vi "Main.vi"() -> ()   [LabVIEW 2017]
uses:
  CTL/REF Channel Select.ctl
  D:/test/ILSTS/LV_IL/LV_IL_Sample_x86/DLL/STSProcess.dll
  DLL/STSProcess.dll
  CTL/Address Cluster.ctl
  D:/test/ILSTS/LV_IL/LV_IL_Sample_x86/DLL/InstrumentDLL.dll
  DLL/InstrumentDLL.dll
  <vilib>/Utility/miscctls.llb/LVStringsAndValuesArrayTypeDef_DBL.ctl
  Share/PowerMonitorType.vi
panel:
  in  "ILSTS":refnum<k24>
  in  "btnzeroing":bool
  in  "btnreadref_data":bool
  in  "btnsaveRawdata":bool
  in  "btnsaveref_rawdata":bool
  in  "chkeach_ch":bool
  in  "btnmeas":bool
  in  "btnset":bool
  in  "Range1":bool
  in  "REF Channel Select":T1={"M1S0C1"=TRUE, "M1S0C2"=FALSE, "M1S0C3"=FALSE, "M1S0C4"=FALSE, "M1S1C1"=FALSE, "M1S1C2"=FALSE, "M1S1C3"=FALSE, "M1S1C4"=FALSE, "M1S2C1"=FALSE, "M1S2C2"=FALSE, "M1S2C3"=FALSE, "M1S2C4"=FALSE, "M1S3C1"=FALSE, "M1S3C2"=FALSE, "M1S3C3"=FALSE, "M1S3C4"=FALSE, "M1S4C1"=FALSE, "M1S4C2"=FALSE, "M1S4C3"=FALSE, "M1S4C4"=FALSE, "M2S0C1"=FALSE, "M2S0C2"=FALSE, "M2S0C3"=FALSE, "M2S0C4"=FALSE, "M2S1C1"=FALSE, "M2S1C2"=FALSE, "M2S1C3"=FALSE, "M2S1C4"=FALSE, "M2S2C1"=FALSE, "M2S2C2"=FALSE, "M2S2C3"=FALSE, "M2S2C4"=FALSE, "M2S3C1"=FALSE, "M2S3C2"=FALSE, "M2S3C3"=FALSE, "M2S3C4"=FALSE, "M2S4C1"=FALSE, "M2S4C2"=FALSE, "M2S4C3"=FALSE, "M2S4C4"=FALSE}
  in  "Range2":bool
  in  "Range3":bool
  in  "Range4":bool
  in  "Range5":bool
  in  "btnget_reference":bool
  in  "Address Cluster":T2={"SPU"=refnum, "MPM"=[], "Port_Count"=0.0, "MPM_Count"=0.0, "SPU_Resource"=[], "USB_Resource"=[], "MPM_Communicater"="", "MPM_Count"=0.0, "MPM_Address"=[], "MPM_Portnumber"=[], "SPU_DeviveID"="", "MPM_communcation_method"=[], "TSL_sweepstartwave"=0.0, "TSL_sweepstopwave"=0.0, "TSL_Address"="", "TSL_Communicater"="", "TSL"=refnum, "tsl_communcation_method"=3, "TSL_Portnumber"=0.0} {"tsl_communcation_method" items=["GPIB", "C232C", "TCPIP", "USB"]; "MPM_communcation_method" items=["GPIB", "C232C", "TCPIP", "USB"]}
  in  "Active Sensors":bool[](array[boolean])
  out "Meas_rang":i32[](array[numeric])
  out "Flag_213":bool
  out "Flag_215":bool
  out "Mergedata_struct":refnum<k24>[](array[refnum])
  out "Meas_monitor_struct":refnum<k24>[](array[refnum])
  out "Ref_monitordata_struct":refnum<k24>[](array[refnum])
  out "Refdata_struct":refnum<k24>[](array[refnum])
  out "Data_struct":refnum<k24>[](array[refnum])
  in  "txtpower":dbl caption="TSL Power(dBm)"
  in  "cmbspeed":u16(ring) caption="SweepSpeed(nm/sec)" items=["1"=1, "2"=5, "5"=10, "10"=20, "20"=40, "50"=50, "100"=80, "200"=100]
  in  "txtstepwave":dbl caption="WavelengthStep(nm)"
  in  "txtstopwave":dbl caption="StopWavelength(nm)"
  in  "txtstartwave":dbl caption="StartWavelength(nm)"
  # "Measurement ch"
  # "Measurement Range"
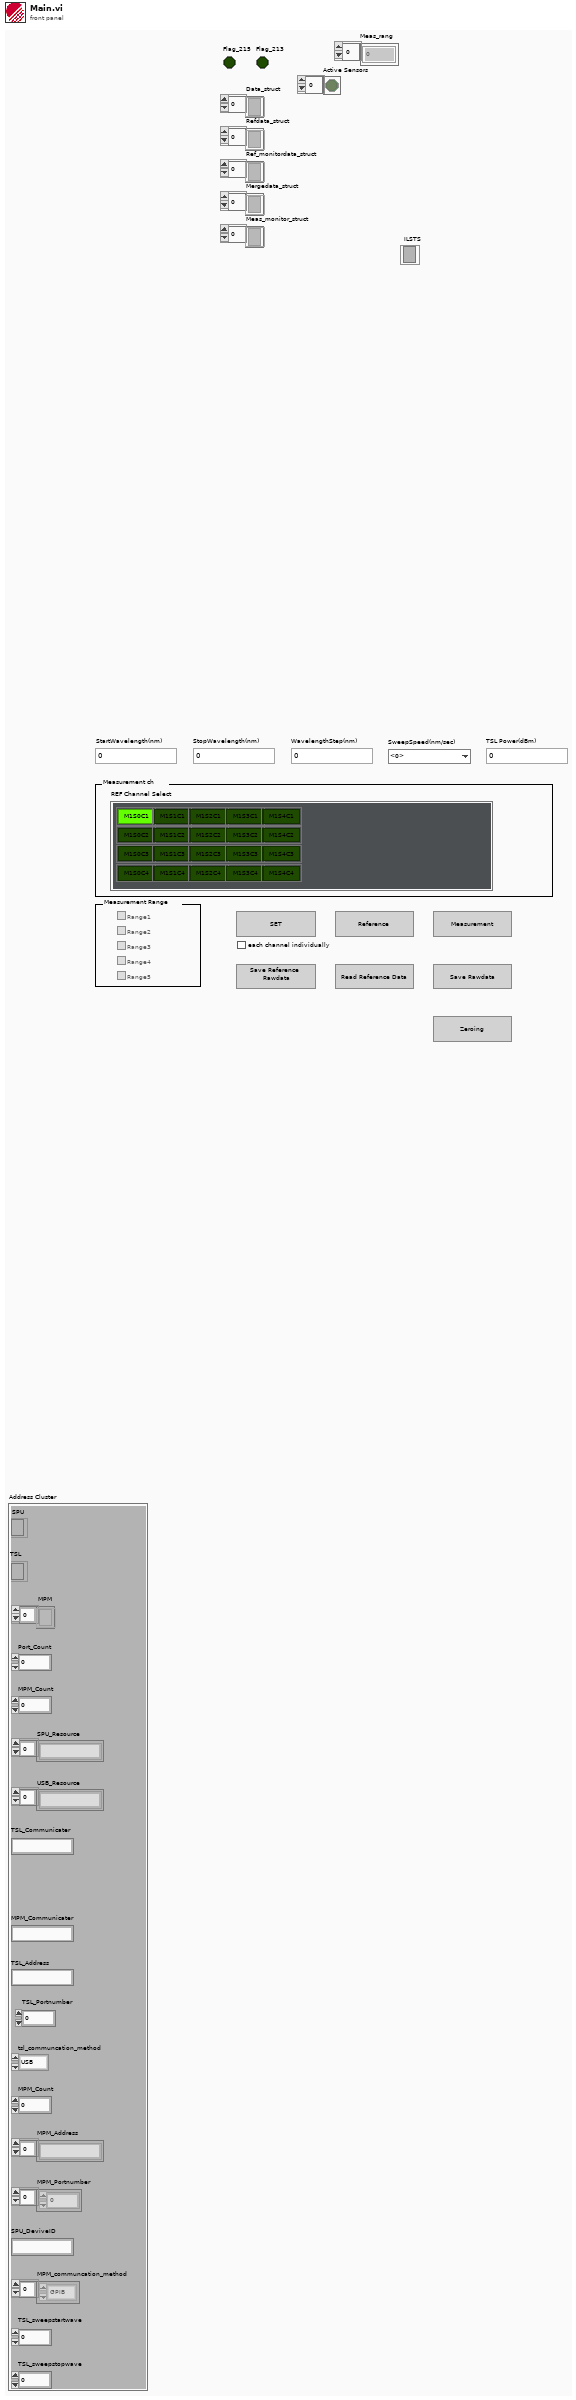
[diagram p1: front panel]
types:
  T1 = typedef "REF Channel Select.ctl" = cluster{"M1S0C1":bool, "M1S0C2":bool, "M1S0C3":bool, "M1S0C4":bool, "M1S1C1":bool, "M1S1C2":bool, "M1S1C3":bool, "M1S1C4":bool, "M1S2C1":bool, "M1S2C2":bool, "M1S2C3":bool, "M1S2C4":bool, "M1S3C1":bool, "M1S3C2":bool, "M1S3C3":bool, "M1S3C4":bool, "M1S4C1":bool, "M1S4C2":bool, "M1S4C3":bool, "M1S4C4":bool, "M2S0C1":bool, "M2S0C2":bool, "M2S0C3":bool, "M2S0C4":bool, "M2S1C1":bool, "M2S1C2":bool, "M2S1C3":bool, "M2S1C4":bool, "M2S2C1":bool, "M2S2C2":bool, "M2S2C3":bool, "M2S2C4":bool, "M2S3C1":bool, "M2S3C2":bool, "M2S3C3":bool, "M2S3C4":bool, "M2S4C1":bool, "M2S4C2":bool, "M2S4C3":bool, "M2S4C4":bool}
  T2 = typedef "Address Cluster.ctl" = cluster{"SPU":refnum<k24>, "MPM":refnum<k24>[], "Port_Count":dbl, "MPM_Count":dbl, "SPU_Resource":string[], "USB_Resource":string[], "MPM_Communicater":string, "MPM_Count":dbl, "MPM_Address":string[], "MPM_Portnumber":dbl[], "SPU_DeviveID":string, "MPM_communcation_method":i32[], "TSL_sweepstartwave":dbl, "TSL_sweepstopwave":dbl, "TSL_Address":string, "TSL_Communicater":string, "TSL":refnum<k24>, "tsl_communcation_method":i32, "TSL_Portnumber":dbl}
  T3 = enum8{"Enabled", "Disabled", "Disabled and Grayed Out"}
  T4 = typedef "LVStringsAndValuesArrayTypeDef_DBL.ctl" = cluster{"String":string, "Value":dbl}[]
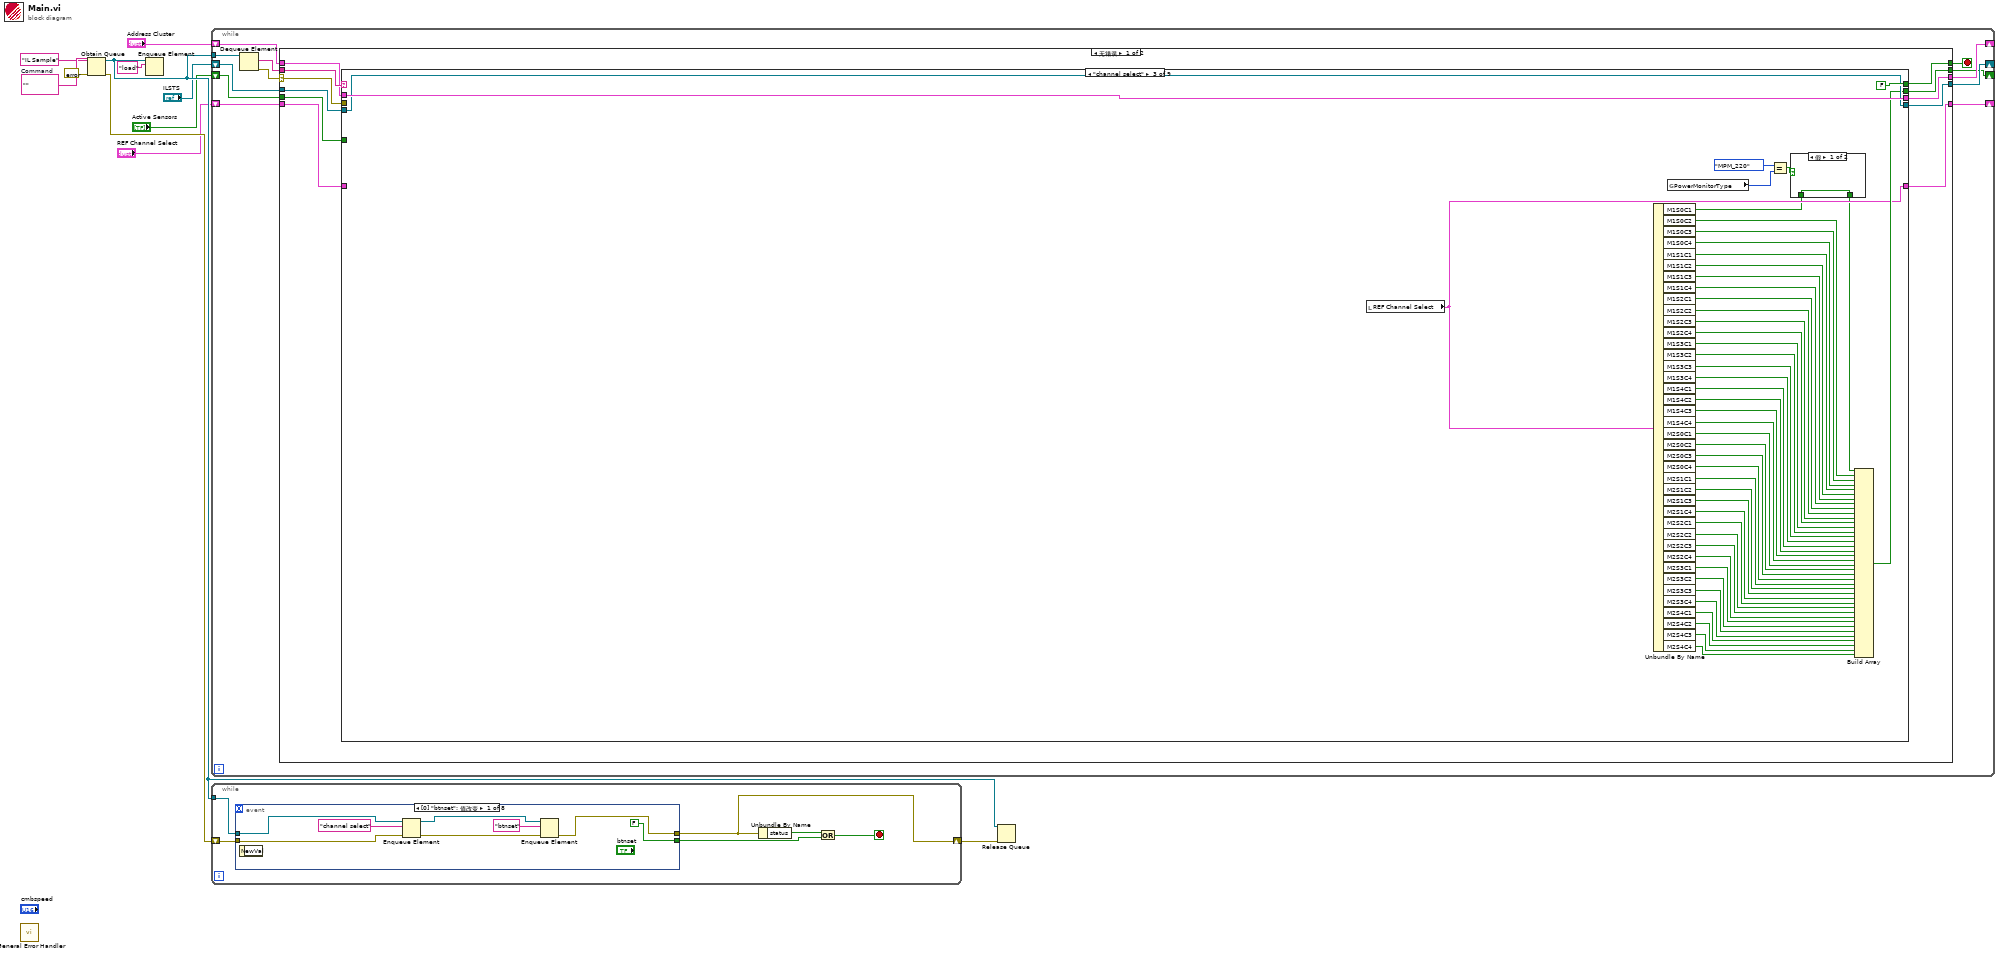
[diagram p0: block diagram]
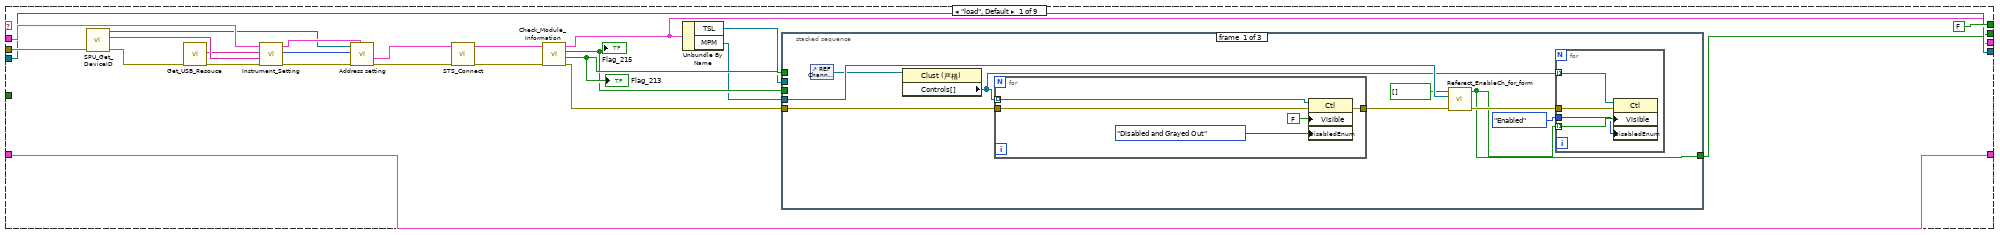
[diagram p2: hidden frame]
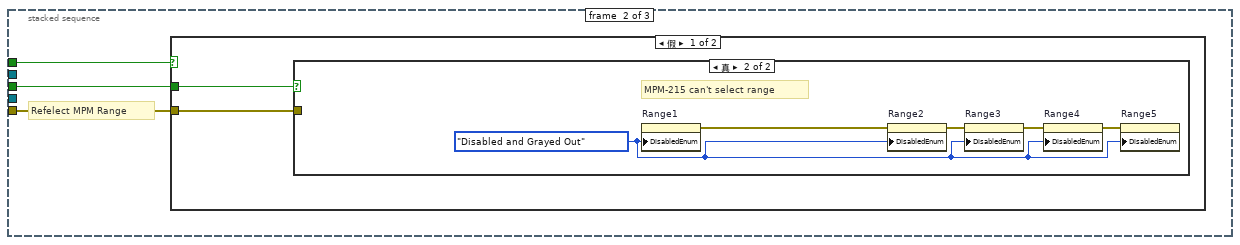
[diagram p3: hidden frame]
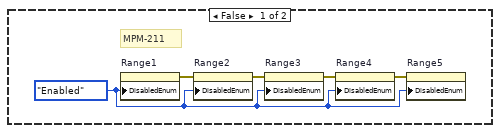
[diagram p4: hidden frame]
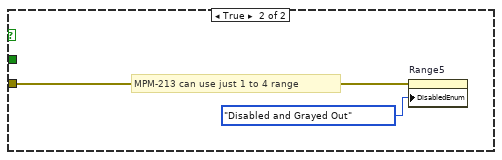
[diagram p5: hidden frame]
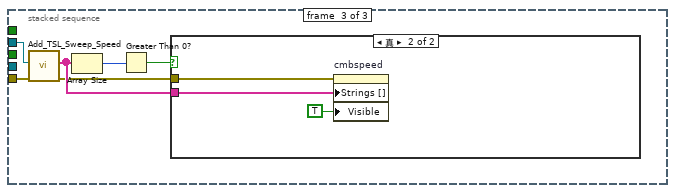
[diagram p6: hidden frame]
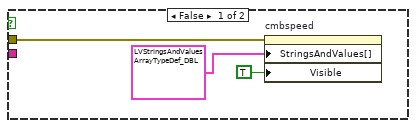
[diagram p7: hidden frame]
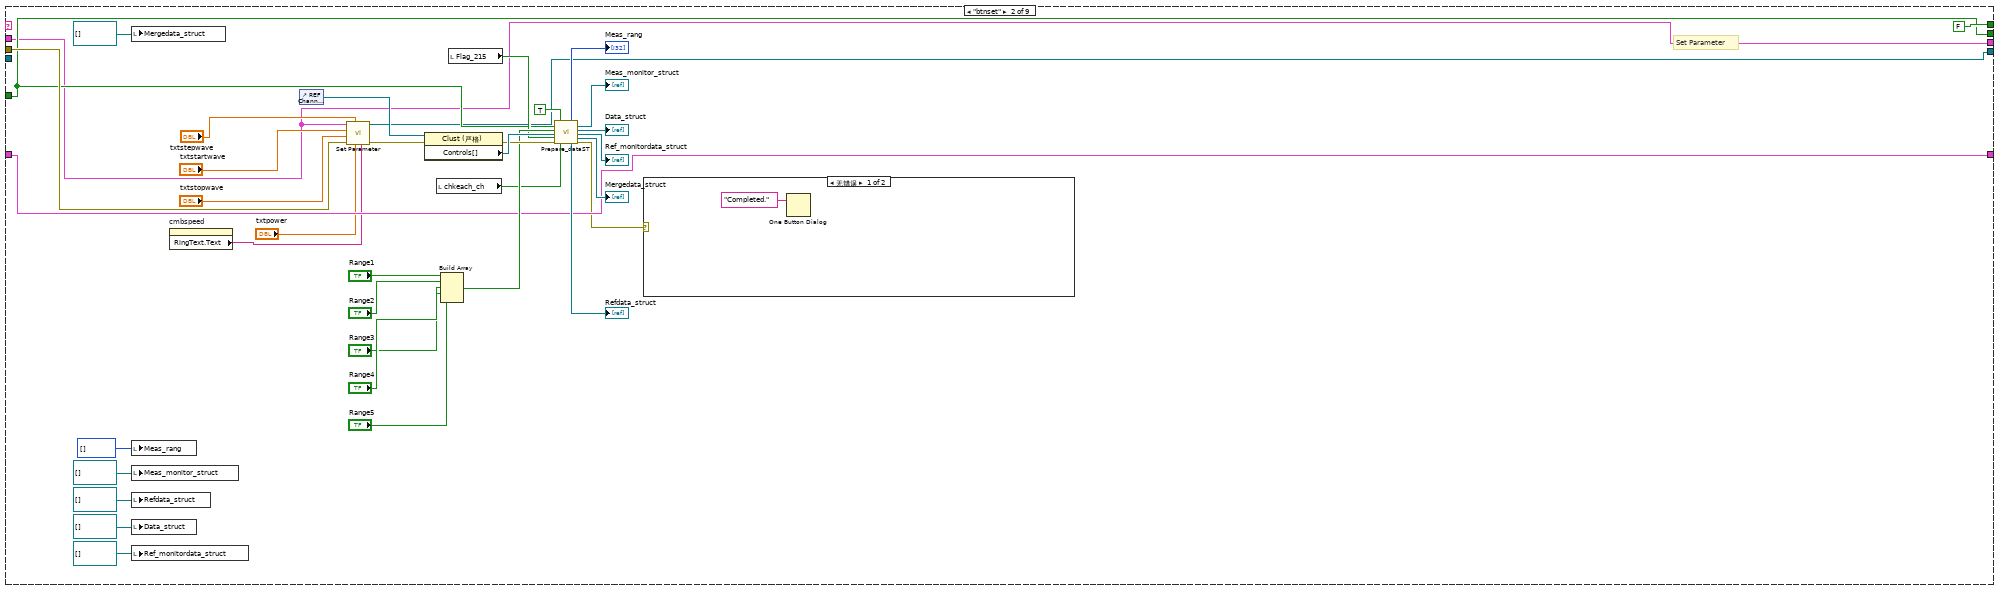
[diagram p8: hidden frame]
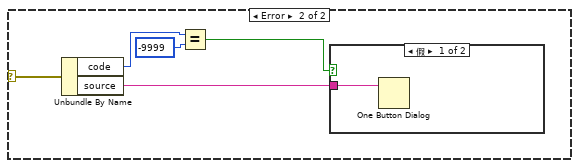
[diagram p9: hidden frame]
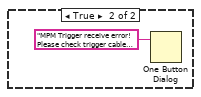
[diagram p10: hidden frame]
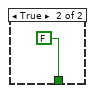
[diagram p11: hidden frame]
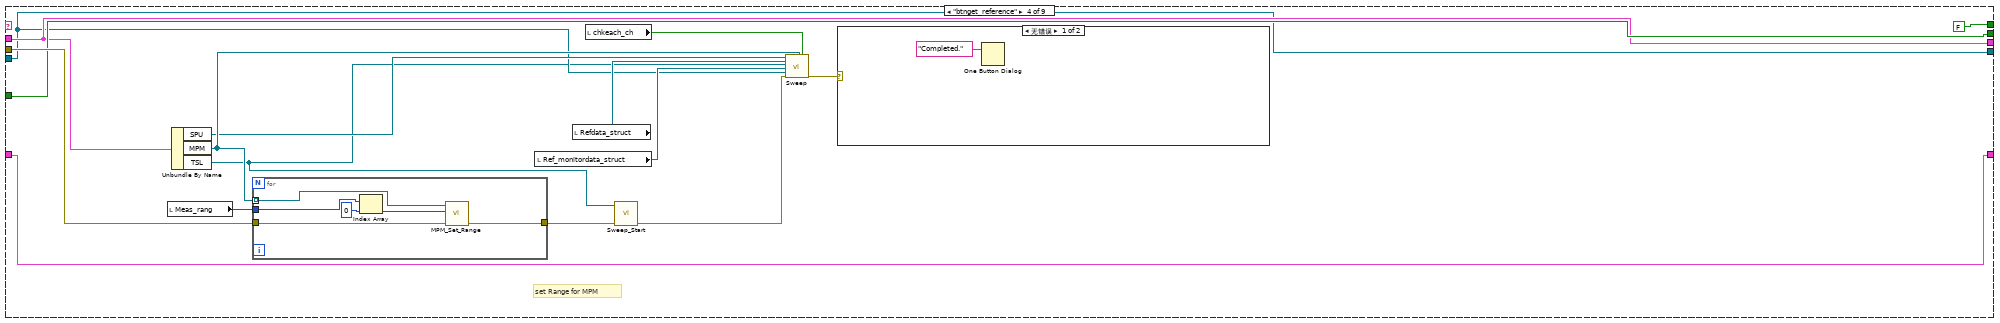
[diagram p12: hidden frame]
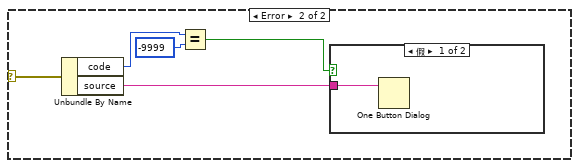
[diagram p13: hidden frame]
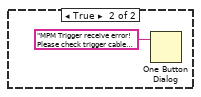
[diagram p14: hidden frame]
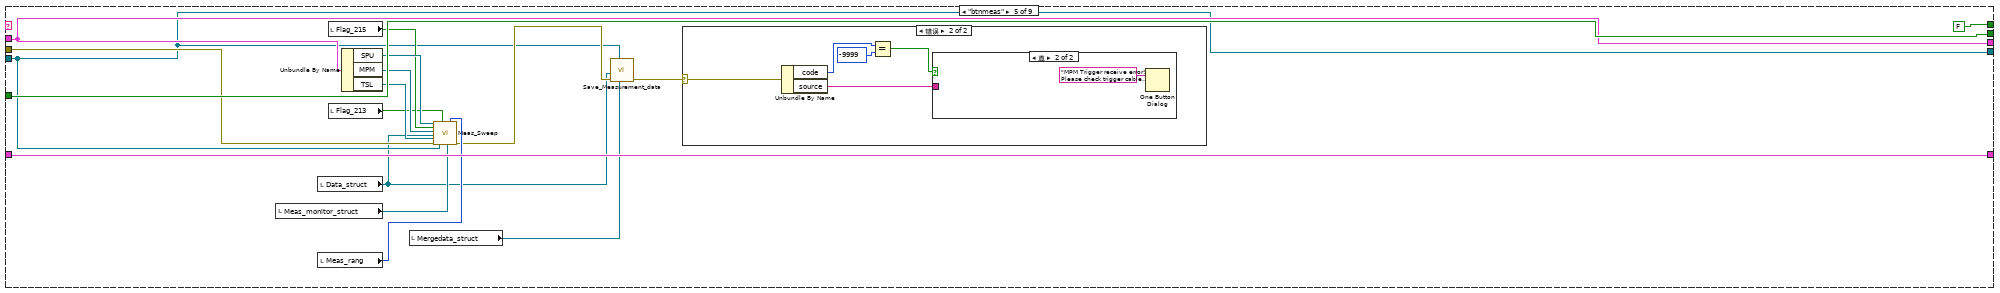
[diagram p15: hidden frame]
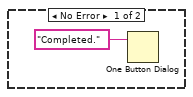
[diagram p16: hidden frame]
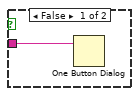
[diagram p17: hidden frame]
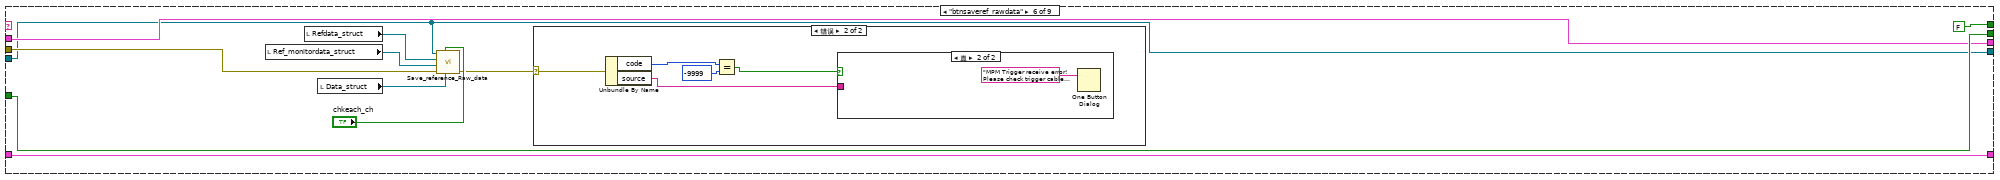
[diagram p18: hidden frame]
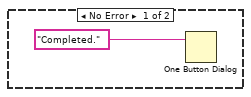
[diagram p19: hidden frame]
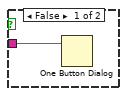
[diagram p20: hidden frame]
diagram:
  w11 = ""  # Command
  n1 = call <vilib>:"General Error Handler.vi"() -> ()  [unwired: 11 in, 5 out]
  n2 = Obtain Queue(name (unnamed)="IL Sample" ("名称（未命名）"), element data type=w11, error in (no error)=errorcluster {"status"=FALSE, "code"=0, "source"=""} ("错误输入（无错误）")) -> (queue out=w6:refnum<queue>, error out=w8:errorcluster)  [unwired: 2 in, 1 out]
  n3 = Enqueue Element(queue=w6, element="load" ("元素")) -> ()  [unwired: 2 in, 3 out]
  n4 = while {
    tunnel: w6 -> [w22]
    shift-right: [w18] -> _
    shift-left: "Address Cluster" -> [w19]
    shift-right: [w16] -> _
    shift-left: "ILSTS" -> [w17]
    shift-right: [w15] -> _
    shift-left: "Active Sensors" -> [w14]
    shift-right: [w12] -> _
    shift-left: "REF Channel Select" -> [w13]
    stop <- w20 stop-if-true
    n5 = Dequeue Element(queue=w22) -> (element=w21:string, error out=w23:errorcluster)  [unwired: 2 in, 2 out]
    n6 = case shown="无错误" w23 {
      selector: w23 -> [w31 _]
      tunnel: w21 -> [w34 _]
      tunnel: [w33 TRUE] -> w20
      tunnel: w19 -> [w32 w334]
      tunnel: [w26 w334] -> w18
      tunnel: w17 -> [w30 w332]
      tunnel: [w29 w332] -> w16
      tunnel: [w28 w333] -> w15
      tunnel: w14 -> [w27 w333]
      tunnel: w13 -> [w25 w331]
      tunnel: [w24 w331] -> w12
      frame No Error {
        n7 = case shown="\"channel select\"" w34 {
          tunnel: [FALSE FALSE FALSE FALSE FALSE FALSE FALSE FALSE FALSE] -> w33
          tunnel: w32 -> [w58 w108 w198 w208 w247 w266 w284 w297 w320]
          tunnel: [w36 w108 w198 w208 w247 w266 w284 w297 w320] -> w26
          tunnel: w31 -> [w57 w122 _ w216 w245 w264 w282 w295 w314]
          tunnel: w30 -> [w44 _ w197 w203 w233 w260 w278 w298 w318]
          tunnel: [w44 w107 w197 w203 w233 w260 w278 w298 w318] -> w29
          tunnel: [w43 w121 w157 w209 w248 w267 w285 w301 w315] -> w28
          tunnel: w27 -> [_ w121 _ w209 w248 w267 w285 w301 w315]
          tunnel: w25 -> [w38 w120 _ w206 w244 w263 w281 w299 w321]
          tunnel: [w38 w120 w156 w206 w244 w263 w281 w299 w321] -> w24
          frame "load", Default {
            n8 = call "SPU_Get_DeviceID.vi"("错误输入（无错误）"=w57) -> ("error IO"=w54:errorcluster, "id"=w55:string[], "引用输出"=w49:refnum<k24>)  [unwired: 7 in]
            n9 = call "Get_USB_Resouce.vi"("error in (no error)"=w54) -> ("error out"=w48:errorcluster, "Get_USB_Resouce"=w53:string[])  [unwired: 8 in, 1 out]
            n10 = call "Instrument_Setting.vi"(8:w48, "id"=w55, "Get_USB_Resouce"=w53, "Address Cluster"=w58) -> ("错误输出"=w47:errorcluster, "PowerMonitorType"=w35:enum16{"DAQ", "MPM_220", "TSL_LOGG"}, "Address Cluster out"=w52:T2)  [unwired: 5 in]
            n11 = call "Address setting.vi"("Address Cluster out输入"=w52, "错误输入（无错误）"=w47, "PowerMonitorType"=w35, "SPU in"=w49) -> ("error out"=w46:errorcluster, "Address Cluster out输出"=w51:T2)  [unwired: 6 in]
            n12 = call "STS_Connect.vi"("error in"=w46, "Address Cluster out输入"=w51) -> ("error out"=w45:errorcluster, "Address Cluster out"=w50:T2)  [unwired: 8 in]
            n13 = call "Check_Module_Information.vi"("Address Cluster"=w50, "错误输入（无错误）"=w45) -> ("Address Cluster out"=w36:T2, "Flag_215"=w41:bool, "Flag_213"=w42:bool, "error out"=w40:errorcluster)  [unwired: 5 in]
            "Flag_215" <- w41
            "Flag_213" <- w42
            n14 = Unbundle By Name(w36) -> ("TSL"=w39:refnum<k24>, "MPM"=w37:refnum<k24>[])
            n15 = stacked-sequence {
              tunnel: w37 -> [w67 _ _]
              tunnel: [w62 _ _] -> w43
              tunnel: w42 -> [_ w79 _]
              tunnel: w41 -> [_ w78 _]
              tunnel: w40 -> [w60 w77 w94]
              tunnel: w39 -> [_ _ w99]
              frame #0 {
                n16 = control-ref of="REF Channel Select"() -> (w65:refnum<vi>)
                n17 = property on="Property Node" class="Clust (严格)"(reference=w65) -> ("Controls[]"=w61:refnum<vi>[])  [unwired: 1 in, 2 out]
                n18 = for {
                  tunnel: w61 -> [w72] mode=indexing
                  tunnel: w60 -> [w71]
                  tunnel: [w70] -> w59
                  n19 = property on="Property Node" class="Ctl"(reference=w72, error in=w71, "Visible"=FALSE ("可见"), "DisabledEnum"=T3."Disabled and Grayed Out" ("禁用")) -> (error out=w70:errorcluster)  [unwired: 1 out]
                }
                n20 = call "Referect_EnableCh_for_form.vi"("错误输入（无错误）"=w59, "MPM"=w67, "数组输入"=bool[] []) -> ("error IO"=w63:errorcluster, "数组输出"=w62:bool[])  [unwired: 7 in]
                n21 = for {
                  tunnel: w61 -> [w76] mode=indexing
                  tunnel: w62 -> [w75] mode=indexing
                  tunnel: T3."Enabled" ("禁用") -> [w74]
                  tunnel: w63 -> [w73]
                  n22 = property on="Property Node" class="Ctl"(reference=w76, error in=w73, "Visible"=w75, "DisabledEnum"=w74) -> ()  [unwired: 2 out]
                }
              }
              frame #1 {
                # "Refelect MPM Range"
                n23 = case shown="假" w79 {
                  tunnel: w78 -> [w81 _]
                  tunnel: w77 -> [w80 w92]
                  frame False {
                    n24 = case shown="真" w81 {
                      tunnel: w80 -> [_ _]
                      frame False {
                        w82 = T3."Enabled" ("禁用")
                        # "MPM-211"
                        n25 = property on="Range1" class="Bool (严格)"("DisabledEnum"=w82) -> (error out=w86:errorcluster)  [unwired: 2 in, 1 out]
                        n26 = property on="Range2" class="Bool (严格)"(error in=w86, "DisabledEnum"=w82) -> (error out=w85:errorcluster)  [unwired: 1 in, 1 out]
                        n27 = property on="Range3" class="Bool (严格)"(error in=w85, "DisabledEnum"=w82) -> (error out=w84:errorcluster)  [unwired: 1 in, 1 out]
                        n28 = property on="Range4" class="Bool (严格)"(error in=w84, "DisabledEnum"=w82) -> (error out=w83:errorcluster)  [unwired: 1 in, 1 out]
                        n29 = property on="Range5" class="Bool (严格)"(error in=w83, "DisabledEnum"=w82) -> ()  [unwired: 1 in, 2 out]
                      }
                      frame True {
                        w87 = T3."Disabled and Grayed Out" ("禁用")
                        # "MPM-215 can't select range"
                        n30 = property on="Range1" class="Bool (严格)"("DisabledEnum"=w87) -> (error out=w91:errorcluster)  [unwired: 2 in, 1 out]
                        n31 = property on="Range2" class="Bool (严格)"(error in=w91, "DisabledEnum"=w87) -> (error out=w90:errorcluster)  [unwired: 1 in, 1 out]
                        n32 = property on="Range3" class="Bool (严格)"(error in=w90, "DisabledEnum"=w87) -> (error out=w89:errorcluster)  [unwired: 1 in, 1 out]
                        n33 = property on="Range4" class="Bool (严格)"(error in=w89, "DisabledEnum"=w87) -> (error out=w88:errorcluster)  [unwired: 1 in, 1 out]
                        n34 = property on="Range5" class="Bool (严格)"(error in=w88, "DisabledEnum"=w87) -> ()  [unwired: 1 in, 2 out]
                      }
                    }
                  }
                  frame True {
                    # "MPM-213 can use just 1 to 4 range"
                    n35 = property on="Range5" class="Bool (严格)"(error in=w92, "DisabledEnum"=T3."Disabled and Grayed Out" ("禁用")) -> ()  [unwired: 1 in, 2 out]
                  }
                }
              }
              frame #2 {
                n36 = call "Add_TSL_Sweep_Speed.vi"("TSL"=w99, "error in (no error)"=w94) -> ("数组输出"=w96:string[], "error out"=w95:errorcluster)  [unwired: 7 in]
                n37 = Array Size(array=w96) -> (size(s)=w98:i32)
                n38 = Greater Than 0?(x=w98) -> (x > 0?=w97:bool)
                n39 = case shown="真" w97 {
                  tunnel: w95 -> [w101 w104]
                  tunnel: w96 -> [_ w103]
                  frame False {
                    n40 = property on="cmbspeed" class="Ring (严格)"(error in=w101, "StringsAndValues[]"=T4 [{"String"="1", "Value"=1.0}, {"String"="5", "Value"=5.0}, {"String"="10", "Value"=10.0}, {"String"="20", "Value"=20.0}, {"String"="40", "Value"=40.0}, {"String"="50", "Value"=50.0}, {"String"="80", "Value"=80.0}, {"String"="100", "Value"=100.0}] ("Strings And Values []"), "Visible"=TRUE ("可见")) -> ()  [unwired: 1 in, 2 out]
                  }
                  frame True {
                    n41 = property on="cmbspeed" class="Ring (严格)"(error in=w104, "Strings []"=w103, "Visible"=TRUE ("可见")) -> ()  [unwired: 1 in, 2 out]
                  }
                }
              }
            }
          }
          frame "btnset" {
            # "Set Parameter"
            n42 = local write "Mergedata_struct"(refnum<k24>[] [] ("Mergedata_struct")) -> ()
            n43 = local write "Meas_rang"(i32[] [] ("Meas_rang")) -> ()
            n44 = local write "Meas_monitor_struct"(refnum<k24>[] [] ("Meas_monitor_struct")) -> ()
            n45 = local write "Refdata_struct"(refnum<k24>[] [] ("Refdata_struct")) -> ()
            n46 = local write "Data_struct"(refnum<k24>[] [] ("Data_struct")) -> ()
            n47 = local write "Ref_monitordata_struct"(refnum<k24>[] [] ("Ref_monitordata_struct")) -> ()
            n48 = property on="cmbspeed" class="Ring (严格)"() -> ("RingText.Text"=w110:string)  [unwired: 2 in, 2 out]
            n49 = control-ref of="REF Channel Select"() -> (w141:refnum<vi>)
            n50 = call "Set Parameter.vi"("RingText.Text"=w110, "txtpower"="txtpower", "txtstepwave"="txtstepwave", "error in"=w122, "txtstopwave"="txtstopwave", "txtstartwave"="txtstartwave", "Address Cluster"=w108) -> ("error out"=w109:errorcluster, "ILSTS"=w107:refnum<k24>)  [unwired: 3 in]
            n51 = property class="Clust (严格)"(reference=w141, error in=w109) -> (error out=w131:errorcluster, "Controls[]"=w132:refnum<vi>[])  [unwired: 1 out]
            n52 = local read "chkeach_ch"() -> (w129:bool)
            n53 = Build Array("Range1", "Range2", "Range3", "Range4", "Range5") -> (w130:bool[])
            n54 = local read "Flag_215"() -> (w128:bool)
            n55 = call "Prepare_dataST.vi"("Active Sensors"=w121, "ranges"=w130, "Controls[]"=w132, "Flag_215"=w128, "error in"=w131, "struct"=TRUE, "chkeach_ch"=w129) -> ("Meas_rang"=→"Meas_rang":i32[], "Refdata_struct"=→"Refdata_struct":refnum<k24>[], "Meas_monitor_struct"=→"Meas_monitor_struct":refnum<k24>[], "Data_struct"=→"Data_struct":refnum<k24>[], "Ref_monitordata_struct"=→"Ref_monitordata_struct":refnum<k24>[], "Mergedata_struct"=→"Mergedata_struct":refnum<k24>[], "error out"=w106:errorcluster)  [unwired: 6 in]
            n56 = case shown="无错误" w106 {
              selector: w106 -> [_ w148]
              frame No Error {
                n57 = One Button Dialog(message="Completed." ("消息")) -> ()  [unwired: 1 in, 1 out]
              }
              frame Error {
                n58 = Unbundle By Name(w148) -> ("code"=w147:i32, "source"=w144:string)
                n59 = Equal?(x=w147, y=-9999) -> (x = y?=w145:bool)
                n60 = case shown="假" w145 {
                  tunnel: w144 -> [w149 _]
                  frame False {
                    n61 = One Button Dialog(message=w149) -> ()  [unwired: 1 in, 1 out]
                  }
                  frame True {
                    n62 = One Button Dialog(message="MPM Trigger receive error! Please check trigger cable connection." ("消息")) -> ()  [unwired: 1 in, 1 out]
                  }
                }
              }
            }
          }
          frame "channel select" {
            n63 = local read "REF Channel Select"() -> (w156:T1)
            n64 = Unbundle By Name(w156) -> ("M1S0C1"=w152:bool, "M1S0C2"=w196:bool, "M1S0C3"=w195:bool, "M1S0C4"=w194:bool, "M1S1C1"=w193:bool, "M1S1C2"=w192:bool, "M1S1C3"=w191:bool, "M1S1C4"=w190:bool, "M1S2C1"=w189:bool, "M1S2C2"=w188:bool, "M1S2C3"=w187:bool, "M1S2C4"=w186:bool, "M1S3C1"=w185:bool, "M1S3C2"=w184:bool, "M1S3C3"=w183:bool, "M1S3C4"=w182:bool, "M1S4C1"=w181:bool, "M1S4C2"=w180:bool, "M1S4C3"=w179:bool, "M1S4C4"=w178:bool, "M2S0C1"=w177:bool, "M2S0C2"=w176:bool, "M2S0C3"=w175:bool, "M2S0C4"=w174:bool, "M2S1C1"=w173:bool, "M2S1C2"=w172:bool, "M2S1C3"=w171:bool, "M2S1C4"=w170:bool, "M2S2C1"=w169:bool, "M2S2C2"=w168:bool, "M2S2C3"=w167:bool, "M2S2C4"=w166:bool, "M2S3C1"=w165:bool, "M2S3C2"=w164:bool, "M2S3C3"=w163:bool, "M2S3C4"=w162:bool, "M2S4C1"=w161:bool, "M2S4C2"=w160:bool, "M2S4C3"=w159:bool, "M2S4C4"=w158:bool)
            n65 = global read "PowerMonitorType.vi" "PowerMonitorType"() -> (w151:enum16{"DAQ", "MPM_220", "TSL_LOGG"})
            n66 = Equal?(x=enum16{"DAQ", "MPM_220", "TSL_LOGG"}."MPM_220", y=w151) -> (x = y?=w154:bool)
            n67 = case shown="假" w154 {
              tunnel: [w200 FALSE] -> w153
              tunnel: w152 -> [w200 _]
              frame False {
              }
              frame True {
              }
            }
            n68 = Build Array(w153, w196, w195, w194, w193, w192, w191, w190, w189, w188, w187, w186, w185, w184, w183, w182, w181, w180, w179, w178, w177, w176, w175, w174, w173, w172, w171, w170, w169, w168, w167, w166, w165, w164, w163, w162, w161, w160, w159, w158) -> (w157:bool[])
          }
          frame "btnget_reference" {
            # "set Range for MPM"
            n69 = local read "Meas_rang"() -> (w217:i32[])
            n70 = Unbundle By Name(w208) -> ("SPU"=w213:refnum<k24>, "MPM"=w214:refnum<k24>[], "TSL"=w202:refnum<k24>)
            n71 = for {
              tunnel: w214 -> [w231] mode=indexing
              tunnel: w217 -> [w230]
              tunnel: w216 -> [w227]
              tunnel: [w226] -> w205
              n72 = Index Array(array=w230, index=0 ("索引")) -> (element=w228:i32)
              n73 = call "MPM_Set_Range.vi"("error in (no error)"=w227, "Range All"=w228, ".NET Reference in"=w231) -> ("error out"=w226:errorcluster)  [unwired: 7 in, 1 out]
            }
            n74 = local read "Ref_monitordata_struct"() -> (w210:refnum<k24>[])
            n75 = local read "Refdata_struct"() -> (w211:refnum<k24>[])
            n76 = local read "chkeach_ch"() -> (w215:bool)
            n77 = call "Sweep_Start.vi"("error in (no error)"=w205, ".NET Reference in"=w202) -> ("error out"=w204:errorcluster)  [unwired: 8 in, 1 out]
            n78 = call "Sweep.vi"("SPU"=w213, "Refdata_struct"=w211, "TSL"=w202, "Ref_monitordata_struct"=w210, "ILSTS"=w203, "错误输入（无错误）"=w204, "MPM"=w214, "chkeach_ch"=w215) -> ("错误输出"=w212:errorcluster)  [unwired: 11 in]
            n79 = case shown="无错误" w212 {
              selector: w212 -> [_ w223]
              frame No Error {
                n80 = One Button Dialog(message="Completed." ("消息")) -> ()  [unwired: 1 in, 1 out]
              }
              frame Error {
                n81 = Unbundle By Name(w223) -> ("code"=w222:i32, "source"=w219:string)
                n82 = Equal?(x=w222, y=-9999) -> (x = y?=w220:bool)
                n83 = case shown="假" w220 {
                  tunnel: w219 -> [w224 _]
                  frame False {
                    n84 = One Button Dialog(message=w224) -> ()  [unwired: 1 in, 1 out]
                  }
                  frame True {
                    n85 = One Button Dialog(message="MPM Trigger receive error! Please check trigger cable connection." ("消息")) -> ()  [unwired: 1 in, 1 out]
                  }
                }
              }
            }
          }
          frame "btnmeas" {
            n86 = local read "Meas_monitor_struct"() -> (w240:refnum<k24>[])
            n87 = local read "Data_struct"() -> (w232:refnum<k24>[])
            n88 = local read "Meas_rang"() -> (w242:i32[])
            n89 = local read "Flag_215"() -> (w238:bool)
            n90 = local read "Flag_213"() -> (w237:bool)
            n91 = Unbundle By Name(w247) -> ("SPU"=w241:refnum<k24>, "MPM"=w239:refnum<k24>[], "TSL"=w243:refnum<k24>)
            n92 = local read "Mergedata_struct"() -> (w234:refnum<k24>[])
            n93 = call "Meas_Sweep.vi"("SPU"=w241, "Flag_215"=w238, "MPM"=w239, "Data_struct"=w232, "TSL"=w243, "错误输入（无错误）"=w245, "ILSTS"=w233, "Flag_213"=w237, "Meas_monitor_struct"=w240, "Meas_rang"=w242) -> ("错误输出"=w236:errorcluster)  [unwired: 9 in]
            n94 = call "Save_Measurement_data.vi"("Mergedata_struct"=w234, "ILSTS"=w233, "错误输入（无错误）"=w236, "Data_struct"=w232) -> ("错误输出"=w235:errorcluster)  [unwired: 7 in]
            n95 = case shown="错误" w235 {
              selector: w235 -> [_ w254]
              frame No Error {
                n96 = One Button Dialog(message="Completed." ("消息")) -> ()  [unwired: 1 in, 1 out]
              }
              frame Error {
                n97 = Unbundle By Name(w254) -> ("code"=w253:i32, "source"=w250:string)
                n98 = Equal?(x=w253, y=-9999) -> (x = y?=w251:bool)
                n99 = case shown="真" w251 {
                  tunnel: w250 -> [w255 _]
                  frame False {
                    n100 = One Button Dialog(message=w255) -> ()  [unwired: 1 in, 1 out]
                  }
                  frame True {
                    n101 = One Button Dialog(message="MPM Trigger receive error! Please check trigger cable connection." ("消息")) -> ()  [unwired: 1 in, 1 out]
                  }
                }
              }
            }
          }
          frame "btnsaveref_rawdata" {
            n102 = local read "Ref_monitordata_struct"() -> (w258:refnum<k24>[])
            n103 = local read "Refdata_struct"() -> (w259:refnum<k24>[])
            n104 = local read "Data_struct"() -> (w261:refnum<k24>[])
            n105 = call "Save_reference_Raw_data.vi"("Data_struct"=w261, "chkeach_ch"="chkeach_ch", "错误输入（无错误）"=w264, "Ref_monitordata_struct"=w258, "Refdata_struct"=w259, "ILSTS"=w260) -> ("错误输出"=w257:errorcluster)  [unwired: 5 in]
            n106 = case shown="错误" w257 {
              selector: w257 -> [_ w273]
              frame No Error {
                n107 = One Button Dialog(message="Completed." ("消息")) -> ()  [unwired: 1 in, 1 out]
              }
              frame Error {
                n108 = Unbundle By Name(w273) -> ("code"=w272:i32, "source"=w269:string)
                n109 = Equal?(x=w272, y=-9999) -> (x = y?=w270:bool)
                n110 = case shown="真" w270 {
                  tunnel: w269 -> [w274 _]
                  frame False {
                    n111 = One Button Dialog(message=w274) -> ()  [unwired: 1 in, 1 out]
                  }
                  frame True {
                    n112 = One Button Dialog(message="MPM Trigger receive error! Please check trigger cable connection." ("消息")) -> ()  [unwired: 1 in, 1 out]
                  }
                }
              }
            }
          }
          frame "btnsaveRawdata" {
            n113 = local read "Meas_monitor_struct"() -> (w276:refnum<k24>[])
            n114 = local read "Data_struct"() -> (w277:refnum<k24>[])
            n115 = local read "Meas_rang"() -> (w280:i32[])
            n116 = call "Save_Raw_data.vi"("Meas_rang"=w280, "错误输入（无错误）"=w282, "Data_struct"=w277, "Meas_monitor_struct"=w276, "ILSTS"=w278) -> ("错误输出"=w279:errorcluster)  [unwired: 6 in]
            n117 = case shown="无错误" w279 {
              selector: w279 -> [_ w291]
              frame No Error {
                n118 = One Button Dialog(message="Completed." ("消息")) -> ()  [unwired: 1 in, 1 out]
              }
              frame Error {
                n119 = Unbundle By Name(w291) -> ("code"=w290:i32, "source"=w287:string)
                n120 = Equal?(x=w290, y=-9999) -> (x = y?=w288:bool)
                n121 = case shown="真" w288 {
                  tunnel: w287 -> [w292 _]
                  frame False {
                    n122 = One Button Dialog(message=w292) -> ()  [unwired: 1 in, 1 out]
                  }
                  frame True {
                    n123 = One Button Dialog(message="MPM Trigger receive error! Please check trigger cable connection." ("消息")) -> ()  [unwired: 1 in, 1 out]
                  }
                }
              }
            }
          }
          frame "btnzeroing" {
            n124 = Unbundle By Name(w297) -> ("MPM"=w296:refnum<k24>[])
            n125 = for {
              tunnel: w296 -> [w304] mode=indexing
              tunnel: w295 -> [w303]
              tunnel: [w302] -> w294
              n126 = call "MPM_Zeroing.vi"("error in (no error)"=w303, ".NET Reference in"=w304) -> ("error out"=w302:errorcluster)  [unwired: 8 in, 1 out]
            }
            n127 = case shown="错误" w294 {
              selector: w294 -> [_ w310]
              frame No Error {
                n128 = One Button Dialog(message="Completed." ("消息")) -> ()  [unwired: 1 in, 1 out]
              }
              frame Error {
                n129 = Unbundle By Name(w310) -> ("code"=w309:i32, "source"=w306:string)
                n130 = Equal?(x=w309, y=-9999) -> (x = y?=w307:bool)
                n131 = case shown="假" w307 {
                  tunnel: w306 -> [w311 _]
                  frame False {
                    n132 = One Button Dialog(message=w311) -> ()  [unwired: 1 in, 1 out]
                  }
                  frame True {
                    n133 = One Button Dialog(message="MPM Trigger receive error! Please check trigger cable connection." ("消息")) -> ()  [unwired: 1 in, 1 out]
                  }
                }
              }
            }
          }
          frame "btnreadref_data" {
            n134 = Unbundle By Name(w320) -> ("TSL"=w319:refnum<k24>)
            n135 = local read "chkeach_ch"() -> (w317:bool)
            n136 = local read "Data_struct"() -> (w316:refnum<k24>[])
            n137 = call "Reference_Data_Read.vi"("Active Sensors"=w315, "chkeach_ch"=w317, "error in"=w314, "ILSTS"=w318, "Data_struct"=w316, "TSL"=w319) -> ("error IO"=w313:errorcluster)  [unwired: 5 in]
            n138 = case shown="错误" w313 {
              selector: w313 -> [_ w328]
              frame No Error {
                n139 = One Button Dialog(message="Completed." ("消息")) -> ()  [unwired: 1 in, 1 out]
              }
              frame Error {
                n140 = Unbundle By Name(w328) -> ("code"=w327:i32, "source"=w324:string)
                n141 = Equal?(x=w327, y=-9999) -> (x = y?=w325:bool)
                n142 = case shown="假" w325 {
                  tunnel: w324 -> [w329 _]
                  frame False {
                    n143 = One Button Dialog(message=w329) -> ()  [unwired: 1 in, 1 out]
                  }
                  frame True {
                    n144 = One Button Dialog(message="MPM Trigger receive error! Please check trigger cable connection." ("消息")) -> ()  [unwired: 1 in, 1 out]
                  }
                }
              }
            }
          }
        }
      }
      frame Error {
      }
    }
  }
  n145 = while {
    tunnel: w6 -> [w340]
    shift-right: [w336] -> w7
    shift-left: w8 -> [w341]
    stop <- w338 stop-if-true
    n146 = event shown="[0] \"btnset\": 值改变" {
      selector: _ -> [_ _ _ _ _ _ _ _]
      dyn-events: _ -> [_ _ _ _ _ _ _ _]
      timeout: _ -> [_ _ _ _ _ _ _ _]
      tunnel: w341 -> [w344 w354 w359 w364 w369 w372 w377 w382]
      tunnel: w340 -> [w345 w353 w358 w363 w368 w370 w375 w380]
      tunnel: [w349 w352 w357 w362 w367 w371 w376 w381] -> w336
      tunnel: [FALSE FALSE FALSE FALSE FALSE FALSE FALSE FALSE] -> w337
      event "btnset": Value Change {
        n147 = event-data() -> ()  [unwired: 1 in, 1 out]
        n148 = Enqueue Element(queue=w345, element="channel select" ("元素"), error in (no error)=w344) -> (queue out=w342:refnum<queue>, error out=w343:errorcluster)  [unwired: 1 in, 1 out]
        n149 = Enqueue Element(queue=w342, element="btnset" ("元素"), error in (no error)=w343) -> (error out=w349:errorcluster)  [unwired: 1 in, 2 out]
      }
      event "btnget_reference": Value Change {
        n150 = event-data() -> ()  [unwired: 1 in, 1 out]
        n151 = Enqueue Element(queue=w353, element="btnget_reference" ("元素"), error in (no error)=w354) -> (error out=w352:errorcluster)  [unwired: 1 in, 2 out]
      }
      event "btnmeas": Value Change {
        n152 = event-data() -> ()  [unwired: 1 in, 1 out]
        n153 = Enqueue Element(queue=w358, element="btnmeas" ("元素"), error in (no error)=w359) -> (error out=w357:errorcluster)  [unwired: 1 in, 2 out]
      }
      event "btnzeroing": Value Change {
        n154 = event-data() -> ()  [unwired: 1 in, 1 out]
        n155 = Enqueue Element(queue=w363, element="btnzeroing" ("元素"), error in (no error)=w364) -> (error out=w362:errorcluster)  [unwired: 1 in, 2 out]
      }
      event "btnsaveref_rawdata": Value Change {
        n156 = event-data() -> ()  [unwired: 1 in, 1 out]
        n157 = Enqueue Element(queue=w368, element="btnsaveref_rawdata" ("元素"), error in (no error)=w369) -> (error out=w367:errorcluster)  [unwired: 1 in, 2 out]
      }
      event Value Change {
        n158 = event-data() -> ()  [unwired: 1 in, 1 out]
        n159 = Enqueue Element(queue=w370, element="channel select" ("元素"), error in (no error)=w372) -> (error out=w371:errorcluster)  [unwired: 1 in, 2 out]
      }
      event "btnreadref_data": Value Change {
        n160 = event-data() -> ()  [unwired: 1 in, 1 out]
        n161 = Enqueue Element(queue=w375, element="btnreadref_data" ("元素"), error in (no error)=w377) -> (error out=w376:errorcluster)  [unwired: 1 in, 2 out]
      }
      event "btnsaveRawdata": Value Change {
        n162 = event-data() -> ()  [unwired: 1 in, 1 out]
        n163 = Enqueue Element(queue=w380, element="btnsaveRawdata" ("元素"), error in (no error)=w382) -> (error out=w381:errorcluster)  [unwired: 1 in, 2 out]
      }
    }
    n164 = Unbundle By Name(w336) -> ("status"=w339:bool)
    n165 = Or(x=w339, y=w337) -> (x .or. y?=w338:bool)
  }
  n166 = Release Queue(queue=w6, error in (no error)=w7) -> ()  [unwired: 1 in, 3 out]
